vi "Make shifts.vi"(0 "startphases":i32=3, 1 "endphases":i32=3, 3 "pulsereps":i32=2 caption="Repetitions", 5 "Durations":dbl[](array[numeric])=[0.2], 6 "Output freq (Hz)":dbl=50.0 format="%#_13g", 7 "randomize":bool=TRUE, 8 "pre cycles":dbl=10.0 caption="Pre cycles", 9 "post cycles":dbl=10.0 caption="Post cycles", 10 "cyclespershift":dbl=10.0 caption="Cycles per pulse", 11 "sinfreq":dbl=1.5 caption="sinefreq", 13 "sinamp":dbl=20.0 caption="sineamp") -> (14 "pulse data":T1, 15 "sine signal":dbl[](array[numeric]), 17 "pulse signal":dbl[](array[numeric]), 18 "totaltime":dbl caption="Total time")   [LabVIEW 2013]
uses:
  Pulse data.ctl
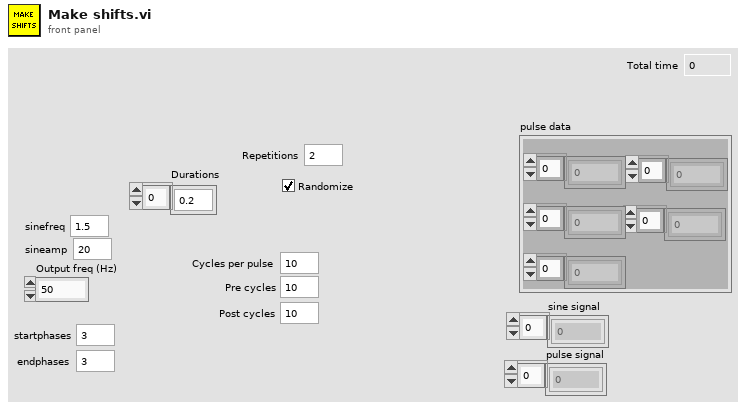
[diagram p1: front panel]
types:
  T1 = typedef "Pulse data.ctl" = cluster{"time":dbl[], "phase":dbl[], "dir/phase2":dbl[], "amplitude":dbl[], "duration":dbl[]}
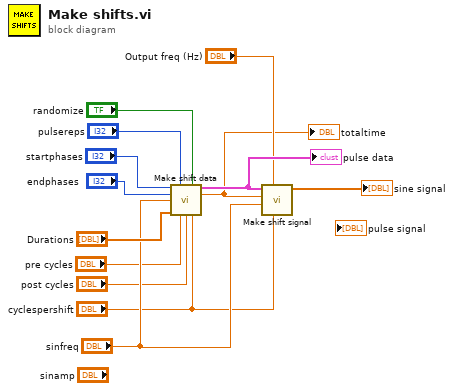
[diagram p0: block diagram]
diagram:
  n1 = call "Make shift data.vi"("startphases"="startphases", "reps"="pulsereps", "randomize"="randomize", "endphases"="endphases", "sinfreq"="sinfreq", "Durations"="Durations", "pre cycles"="pre cycles", "post cycles"="post cycles", "cyclesperpulse"="cyclespershift") -> ("pulse data"=w11:T1, "totaltime"=w6:dbl)  [unwired: 5 in]
  "pulse data" <- w11
  "totaltime" <- w6
  n2 = call "Make shift signal.vi"("cyclesperstim"="cyclespershift", "Output freq (Hz)"="Output freq (Hz)", "sinfreq"="sinfreq", "total time"=w6, "pulse data"=w11) -> ("sine signal"=→"sine signal":dbl[])  [unwired: 6 in]
